vi "MCCETC02_Main.vi"(7 "stop_external":refnum<vi>, 8 "input cluster":T1) -> ()   [LabVIEW 2019]
uses:
  cluster_ref_MCCETC.ctl
panel:
  in  "Logging":bool=TRUE
  out "status_log":bool caption="Status"
  out "T6":dbl format="%.2f"
  out "T5":dbl format="%.2f"
  out "T4":dbl format="%.2f"
  out "T3":dbl format="%.2f"
  out "T2":dbl format="%.2f"
  in  "Tab Control":enum32{"IVC & Fridge", "He Lines"}(tab)
  out "T0 Chart":waveform(dbl)[](graph)
  out "T1 Chart":waveform(dbl)[](graph)
  out "T2 Chart":waveform(dbl)[](graph)
  out "T3 Chart":waveform(dbl)[](graph)
  out "T4 Chart":waveform(dbl)[](graph)
  out "T5 Chart":waveform(dbl)[](graph)
  out "T6 Chart":waveform(dbl)[](graph)
  in  "Readout Interval":i32=5 caption="sec"
  in  "units":i32(ring) items=["degC", "degF", "kelvin", "raw"]
  out "T1":dbl format="%.2f"
  out "T0":dbl format="%.2f"
  out "Readout Status":bool
  out "Last Measured":timestamp format="%<%Y-%m-%d %H:%M:%S>T"
  in  "Stop":bool
  # "MCC E-TC #02:  Thermocouples for Target Chambers & Fill Lines"
  # "IVC Bottom"
  # "IVC Top"
  # "Fridge Top"
  # "LHe FL Stinger"
  # "LHe FL #1"
  # "LHe FL #2"
  # "Sep. Line"
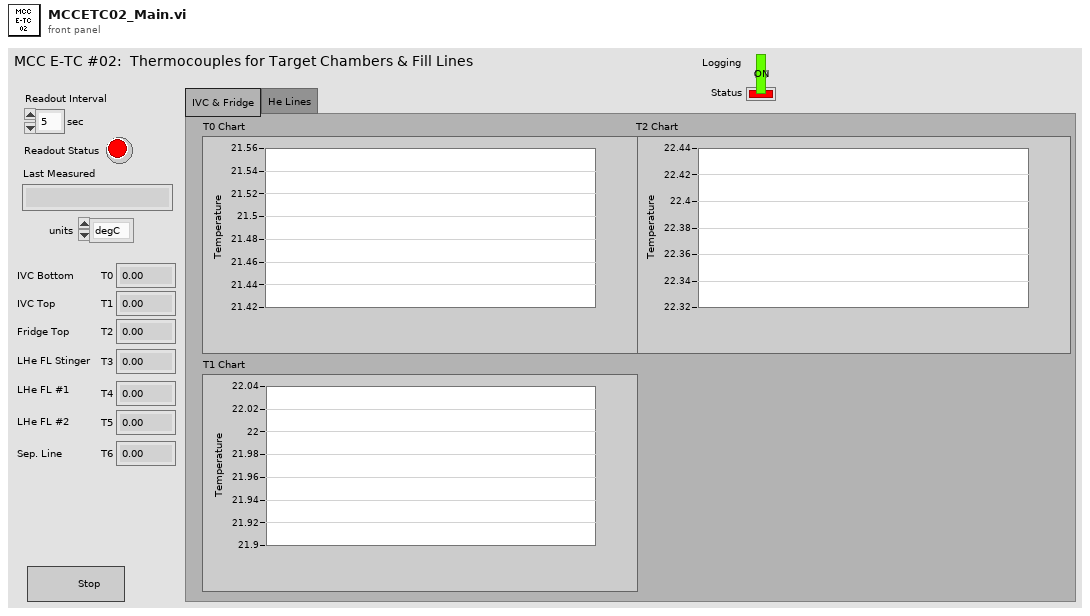
[diagram p1: front panel]
types:
  T1 = typedef "cluster_ref_MCCETC.ctl" = cluster{"Status":refnum<vi>, "T":refnum<vi>[]}
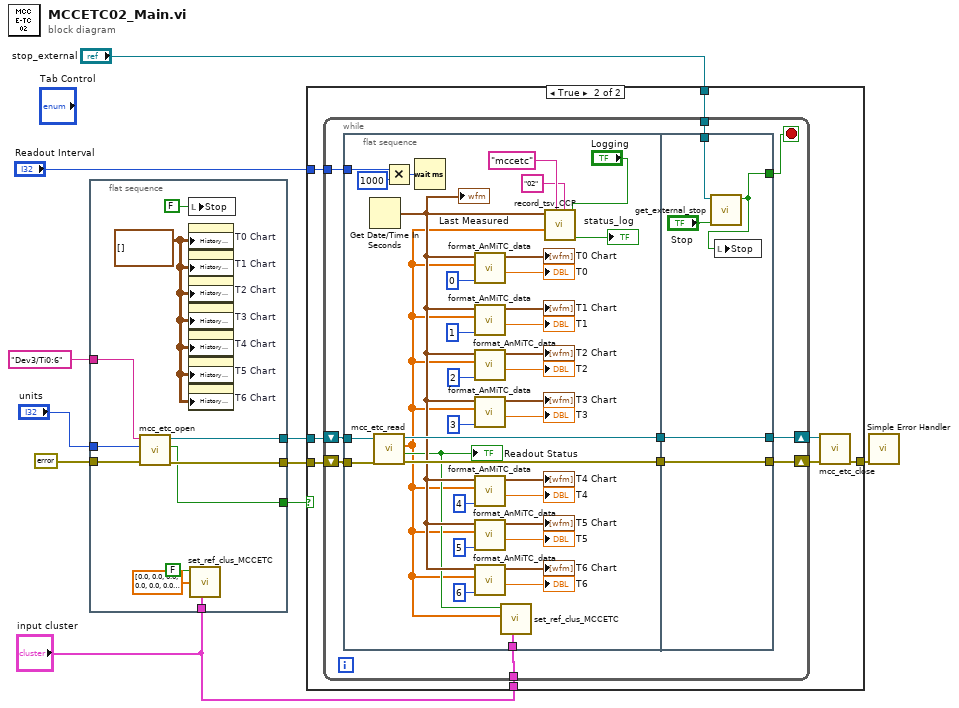
[diagram p0: block diagram]
diagram:
  n1 = flat-sequence {
    tunnel: [w21] -> w10
    tunnel: errorcluster {"status"=FALSE, "code"=0, "source"=""} ("error in") -> [w20]
    tunnel: [w19] -> w8
    tunnel: "Dev3/Ti0:6" ("Device/Channel Name") -> [w18]
    tunnel: "units" -> [w17]
    tunnel: [w16] -> w3
    tunnel: "input cluster" -> [w15]
    frame #0 {
      w11 = waveform(dbl)[][] [] ("History Data")
      n2 = call "mcc_etc_open.vi"("error in"=w20, "units"=w17, "name"=w18) -> ("error out"=w19:errorcluster, "status"=w16:bool, "task out"=w21:refnum<k24>)  [unwired: 6 in]
      n3 = local write "Stop"(FALSE ("Stop")) -> ()
      n4 = property on="T0 Chart" class="WFChart (strict)"("History Data"=w11) -> ()  [unwired: 2 in, 2 out]
      n5 = property on="T1 Chart" class="WFChart (strict)"("History Data"=w11) -> ()  [unwired: 2 in, 2 out]
      n6 = property on="T2 Chart" class="WFChart (strict)"("History Data"=w11) -> ()  [unwired: 2 in, 2 out]
      n7 = property on="T3 Chart" class="WFChart (strict)"("History Data"=w11) -> ()  [unwired: 2 in, 2 out]
      n8 = property on="T4 Chart" class="WFChart (strict)"("History Data"=w11) -> ()  [unwired: 2 in, 2 out]
      n9 = property on="T5 Chart" class="WFChart (strict)"("History Data"=w11) -> ()  [unwired: 2 in, 2 out]
      n10 = property on="T6 Chart" class="WFChart (strict)"("History Data"=w11) -> ()  [unwired: 2 in, 2 out]
      n11 = call "set_ref_clus_MCCETC.vi"("cluster_ref"=w15, "T"=dbl[] [0.0, 0.0, 0.0, 0.0, 0.0, 0.0, 0.0], "status"=FALSE) -> ()  [unwired: 9 in]
    }
  }
  n12 = case shown="True" w3 {
    tunnel: w10 -> [_ w30]
    tunnel: w8 -> [w22 w29]
    tunnel: "Readout Interval" -> [_ w26]
    tunnel: [w22 w25] -> w4
    tunnel: "input cluster" -> [_ w24]
    tunnel: "stop_external" -> [_ w23]
    frame False {
    }
    frame True {
      n13 = while {
        shift-right: [w38] -> w27
        shift-left: w29 -> [w39]
        shift-right: [w37] -> w28
        shift-left: w30 -> [w40]
        tunnel: w26 -> [w36]
        tunnel: w24 -> [w32]
        tunnel: w23 -> [w31]
        stop <- w33 stop-if-true
        n14 = flat-sequence {
          tunnel: w40 -> [w76]
          tunnel: w39 -> [w75]
          tunnel: w36 -> [w72]
          tunnel: [w74] -> w35
          tunnel: [w73] -> w34
          tunnel: w32 -> [w41]
          tunnel: [w80] -> w37
          tunnel: [w81] -> w38
          tunnel: w35 -> [w81]
          tunnel: w34 -> [w80]
          tunnel: [w78] -> w33
          tunnel: w31 -> [w77]
          frame #0 {
            n15 = Get Date/Time In Seconds() -> (seconds since 1Jan1904=w48:timestamp)
            "Last Measured" <- w48
            n16 = call "mcc_etc_read.vi"("error in"=w75, "task in"=w76) -> ("error out"=w74:errorcluster, "status"=w43:bool, "temperature_array"=w42:dbl[], "task out"=w73:refnum<k24>)  [unwired: 6 in]
            "Readout Status" <- w43
            n17 = Multiply(x=w72, y=1000) -> (x*y=w59:i32)
            n18 = Wait (ms)(milliseconds to wait=w59) -> ()  [unwired: 1 out]
            n19 = call "format_AnMiTC_data.vi"("index"=0, "value_array"=w42, "time"=w48) -> ("value"=→"T0":dbl, "waveform_array"=→"T0 Chart":waveform(dbl)[])  [unwired: 7 in]
            n20 = call "format_AnMiTC_data.vi"("index"=1, "value_array"=w42, "time"=w48) -> ("value"=→"T1":dbl, "waveform_array"=→"T1 Chart":waveform(dbl)[])  [unwired: 7 in]
            n21 = call "format_AnMiTC_data.vi"("index"=2, "value_array"=w42, "time"=w48) -> ("value"=→"T2":dbl, "waveform_array"=→"T2 Chart":waveform(dbl)[])  [unwired: 7 in]
            n22 = call "format_AnMiTC_data.vi"("index"=3, "value_array"=w42, "time"=w48) -> ("value"=→"T3":dbl, "waveform_array"=→"T3 Chart":waveform(dbl)[])  [unwired: 7 in]
            n23 = call "format_AnMiTC_data.vi"("index"=4, "value_array"=w42, "time"=w48) -> ("value"=→"T4":dbl, "waveform_array"=→"T4 Chart":waveform(dbl)[])  [unwired: 7 in]
            n24 = call "format_AnMiTC_data.vi"("index"=5, "value_array"=w42, "time"=w48) -> ("value"=→"T5":dbl, "waveform_array"=→"T5 Chart":waveform(dbl)[])  [unwired: 7 in]
            n25 = call "format_AnMiTC_data.vi"("index"=6, "value_array"=w42, "time"=w48) -> ("value"=→"T6":dbl, "waveform_array"=→"T6 Chart":waveform(dbl)[])  [unwired: 7 in]
            n26 = call "set_ref_clus_MCCETC.vi"("cluster_ref"=w41, "T"=w42, "status"=w43) -> ()  [unwired: 9 in]
            n27 = call "record_tsv_CCP.vi"("logging_on"="Logging", "file_name"="02", "folder_name"="mccetc", "value_array"=w42, "time"=w48) -> ("status"=→"status_log":bool)  [unwired: 5 in, 1 out]
          }
          frame #1 {
            n28 = call "get_external_stop.vi"("stop_internal"="Stop", "ref_stop_external"=w77) -> ("stop_output"=w78:bool)  [unwired: 9 in]
            n29 = local write "Stop"(w78) -> ()
          }
        }
      }
      n30 = call "mcc_etc_close.vi"("error in"=w27, "task in"=w28) -> ("error out"=w25:errorcluster)  [unwired: 8 in, 1 out]
    }
  }
  n31 = call <vilib>:"Simple Error Handler.vi"("error in (no error)"=w4) -> ()  [unwired: 4 in, 5 out]
